vi "FaceLandmark.vi"(7 "model":T1 items=["Large", "Small", "Helen"], 8 "error in (no error)":errorcluster, 9 "FaceLocations":refnum<k24>, 10 "FaceImage":refnum<k24>, 11 "FaceRecognition in":refnum<class "FaceRecognition.lvclass">) -> (0 "error out":errorcluster, 1 "FaceLandmark":refnum<k24>, 2 "FaceImage 2":refnum<k24>, 3 "FaceRecognition out":refnum<class "FaceRecognition.lvclass">)   [LabVIEW 2020, in "FaceRecognitionDotNet.lvlib" / "FaceRecognition.lvclass"]
uses:
  FaceRecognition.lvclass
  dll/FaceRecognitionDotNet.dll
  ctl/LandmarkModel.ctl
  FaceRecognition.lvclass/FaceRecognition.ctl
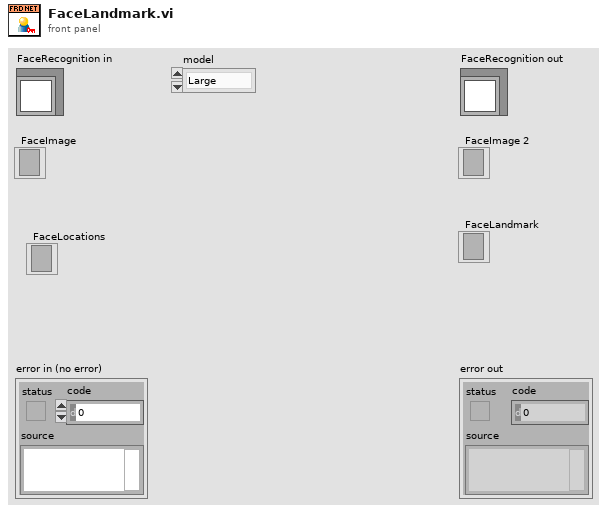
[diagram p1: front panel]
types:
  T1 = typedef "FaceRecognitionDotNet.lvlib/FaceRecognition.lvclass/LandmarkModel.ctl" = i32
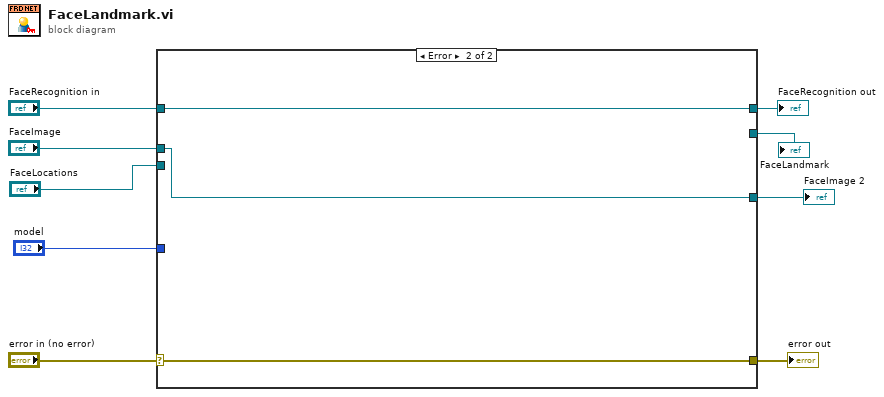
[diagram p0: block diagram]
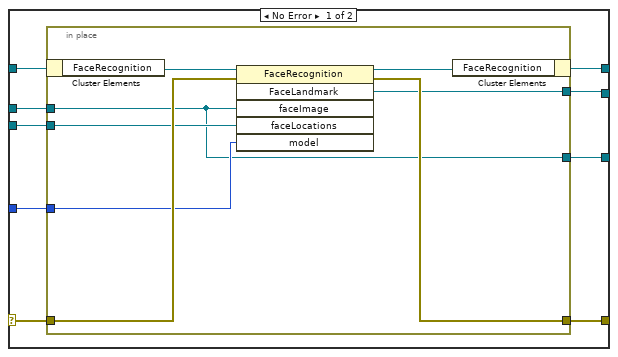
[diagram p2: hidden frame]
diagram:
  n1 = case shown="Error" "error in (no error)" {
    selector: "error in (no error)" -> [w16 w29]
    tunnel: [w15 w29] -> w8
    tunnel: [w17 w28] -> w6
    tunnel: "FaceRecognition in" -> [w18 w28]
    tunnel: [w14 _] -> w3
    tunnel: "FaceImage" -> [w13 w27]
    tunnel: "FaceLocations" -> [w12 _]
    tunnel: "model" -> [w11 _]
    tunnel: [w10 w27] -> w1
    frame No Error {
      n2 = in-place {
        in-place-border: w16 -> [w24]
        in-place-border: [w23] -> w15
        in-place-border: [w22] -> w14
        in-place-border: w13 -> [w19]
        in-place-border: w12 -> [w21]
        in-place-border: w11 -> [w20]
        in-place-border: [w19] -> w10
        n3 = in-place-cluster #1(w18) -> ("FaceRecognition"=w26:refnum<k24>)
        n4 = invoke class="FaceRecognition" method="FaceLandmark"(reference=w26, error in=w24, "faceImage"=w19, "faceLocations"=w21, "model"=w20) -> (reference out=w25:refnum<k24>, error out=w23:errorcluster, "FaceLandmark"=w22:refnum<k24>)  [unwired: 1 in, 3 out]
        n5 = in-place-cluster #1("FaceRecognition"=w25) -> (w17:refnum<class "FaceRecognition.lvclass">)
      }
    }
    frame Error {
    }
  }
  "error out" <- w8
  "FaceRecognition out" <- w6
  "FaceLandmark" <- w3
  "FaceImage 2" <- w1
